vi "Set Values by Cluster.vi"(8 "error in (no error)":errorcluster, 10 "Cluster":variant, 11 "Table in":refnum<class "Basic Table.lvclass">) -> (0 "error out":errorcluster, 3 "Table out":refnum<class "Basic Table.lvclass">)   [LabVIEW 2020, in "Table.lvlib" / "Basic Table.lvclass"]
uses:
  Basic Table.lvclass
  Basic Table.lvclass/Basic Table.ctl
  Table Configuration Interface/Table Configuration Interface.lvclass
  Column Libraries/Column Interface/Column Interface Class/Column Interface.lvclass
  <vilib>/Utility/Data Type/NI_Data Type.lvlib
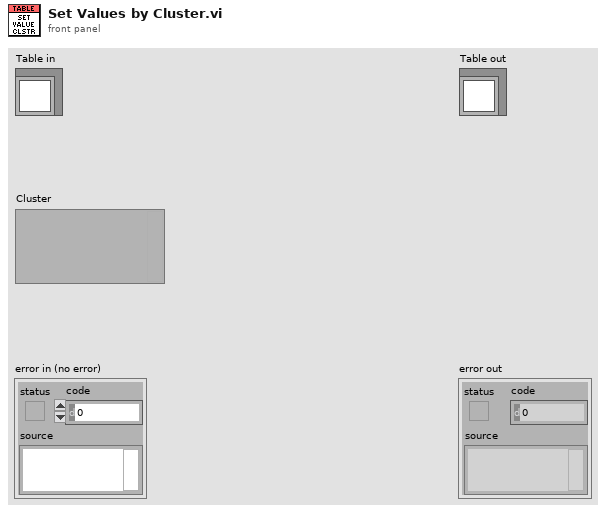
[diagram p1: front panel]
types:
  T1 = map{string, refnum<class "Column Interface.lvclass">}
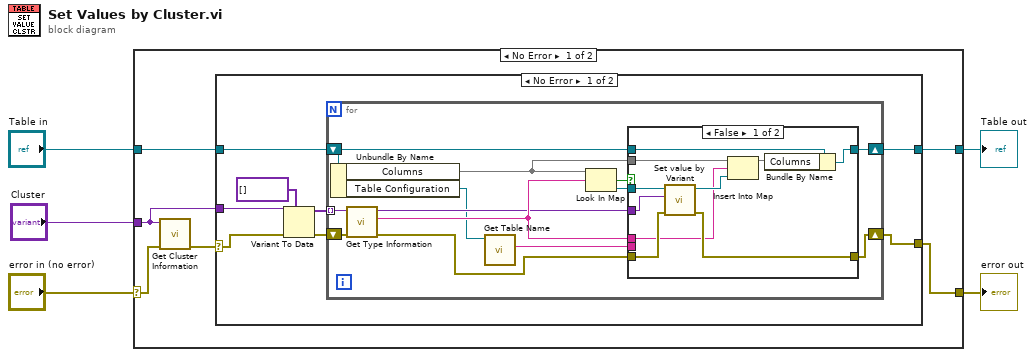
[diagram p0: block diagram]
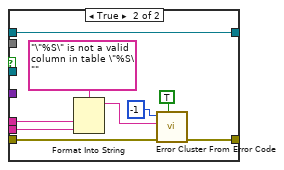
[diagram p2: hidden frame]
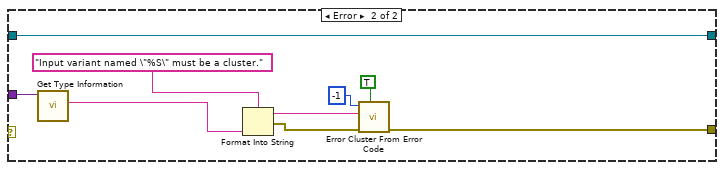
[diagram p3: hidden frame]
diagram:
  n1 = case shown="No Error" "error in (no error)" {
    selector: "error in (no error)" -> [w11 w61]
    tunnel: [w7 w61] -> w4
    tunnel: [w6 w60] -> w2
    tunnel: "Table in" -> [w8 w60]
    tunnel: "Cluster" -> [w9 _]
    frame No Error {
      n2 = call <vilib>:"Get Cluster Information.vi"("error in (no error)"=w11, "variant"=w9) -> ("error out"=w10:errorcluster)  [unwired: 8 in, 1 out]
      n3 = case shown="No Error" w10 {
        selector: w10 -> [w15 _]
        tunnel: w9 -> [w19 w59]
        tunnel: w8 -> [w16 w51]
        tunnel: [w13 w52] -> w7
        tunnel: [w12 w51] -> w6
        frame No Error {
          n4 = Variant To Data(error in=w15, type=variant[] [], Variant=w19) -> (data=w17:variant[], error out=w14:errorcluster)
          n5 = for {
            tunnel: w17 -> [w26] mode=indexing
            shift-right: [w28] -> w13
            shift-left: w14 -> [w29]
            shift-right: [w23] -> w12
            shift-left: w16 -> [w24]
            n6 = Unbundle By Name(w24) -> ("Columns"=w25:T1, "Table Configuration"=w22:refnum<class "Table Configuration Interface.lvclass">)
            n7 = call <vilib>:"Get Type Information.vi"("error in (no error)"=w29, "variant"=w26) -> ("error out"=w20:errorcluster, "name"=w30:string)  [unwired: 5 in, 3 out]
            n8 = call-dynamic "Get Table Name.vi"("Table Configuration Interface in"=w22) -> ("Table Name"=w21:string)  [unwired: 8 in, 2 out]
            n9 = Look In Map(map=w25, key=w30) -> (key not found?=w31:bool, value=w27:refnum<class "Column Interface.lvclass">)  [unwired: 1 in]
            n10 = case shown="False" w31 {
              tunnel: w30 -> [w35 w49]
              tunnel: w21 -> [_ w48]
              tunnel: w20 -> [w39 w44]
              tunnel: [w38 w43] -> w28
              tunnel: w27 -> [w41 _]
              tunnel: w26 -> [w40 _]
              tunnel: w25 -> [w37 _]
              tunnel: w24 -> [w34 w42]
              tunnel: [w32 w42] -> w23
              frame False {
                n11 = call-dynamic "Set value by Variant.vi"("error in (no error)"=w39, "Variant"=w40, "Column Interface in"=w41) -> ("error out"=w38:errorcluster, "Column Interface out"=w36:refnum<class "Column Interface.lvclass">)  [unwired: 7 in]
                n12 = Insert Into Map(map in=w37, key=w35, value=w36) -> (map out=w33:T1)  [unwired: 2 out]
                n13 = Bundle By Name(cluster=w34, "Columns"=w33) -> (w32:refnum<class "Basic Table.lvclass">)
              }
              frame True {
                n14 = Format Into String(format string="\"%S\" is not a valid column in table \"%S\"", w49, w48) -> (resulting string=w47:string)  [unwired: 2 in, 1 out]
                n15 = call <vilib>:"Error Cluster From Error Code.vi"("show call chain? (False)"=TRUE, "error in (no error)"=w44, "error message (\"\")"=w47, "error code (0)"=-1) -> ("error out"=w43:errorcluster)  [unwired: 5 in]
              }
            }
          }
        }
        frame Error {
          n16 = call <vilib>:"Get Type Information.vi"("variant"=w59) -> ("name"=w57:string)  [unwired: 6 in, 4 out]
          n17 = Format Into String(format string="Input variant named \"%S\" must be a cluster.", w57) -> (resulting string=w55:string, error out=w56:errorcluster)  [unwired: 2 in]
          n18 = call <vilib>:"Error Cluster From Error Code.vi"("show call chain? (False)"=TRUE, "error in (no error)"=w56, "error message (\"\")"=w55, "error code (0)"=-1) -> ("error out"=w52:errorcluster)  [unwired: 5 in]
        }
      }
    }
    frame Error {
    }
  }
  "error out" <- w4
  "Table out" <- w2
